vi "Error Handler.vi"(8 "Error code":T1=enum."5005: Path Type Not Supported") -> (0 "error out":errorcluster)   [LabVIEW 2016, in "LV-Data.PGSQL.lvclass"]
uses:
  LV-Data.PGSQL.lvclass
  Typedefs/Errors--enum.ctl
  <vilib>/Utility/error.llb/Error Cluster From Error Code.vi
  <vilib>/ErrorRing/Error Ring.xnode
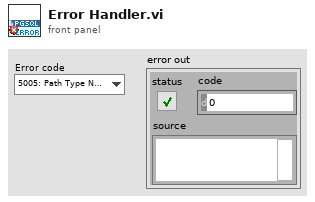
[diagram p1: front panel]
types:
  T1 = typedef "LV-Data.PGSQL.lvclass/Errors--enum.ctl" = enum16{"0: None", "5005: Path Type Not Supported", "5006: Number of Variables", "5008: Cannot write two data points", "5030: Start and End Times Identical", "5031: Input is not wholly", "5033: Bad path or paths", "5040: Invalid Instrument Name", "5050: Column can only hold string", "5051: Column can only hold bool", "5052: Column can only hold double", "5053: Column can only hold int"}
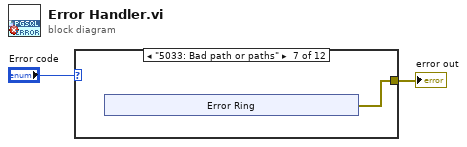
[diagram p0: block diagram]
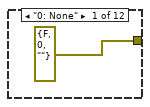
[diagram p2: hidden frame]
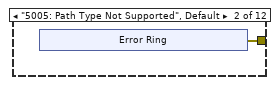
[diagram p3: hidden frame]
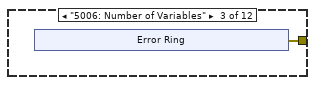
[diagram p4: hidden frame]
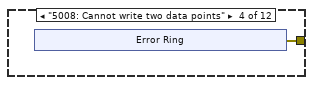
[diagram p5: hidden frame]
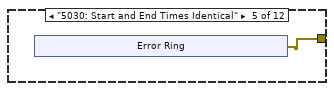
[diagram p6: hidden frame]
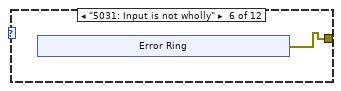
[diagram p7: hidden frame]
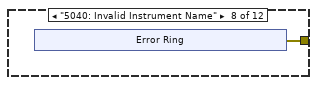
[diagram p8: hidden frame]
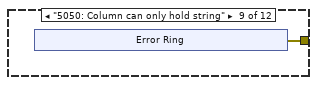
[diagram p9: hidden frame]
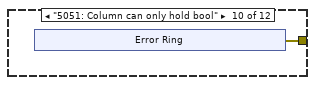
[diagram p10: hidden frame]
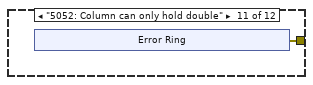
[diagram p11: hidden frame]
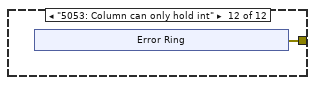
[diagram p12: hidden frame]
diagram:
  n1 = case shown="\"5033: Bad path or paths\"" "Error code" {
    tunnel: [errorcluster {"status"=FALSE, "code"=0, "source"=""} ("error out") w4 w10 w16 w22 w28 w34 w40 w46 w52 w58 w64] -> w1
    frame "0: None" {
    }
    frame "5005: Path Type Not Supported", Default {
      n2 = xnode "Error Ring"() -> ("error out"=w4:errorcluster)
    }
    frame "5006: Number of Variables" {
      n3 = xnode "Error Ring"() -> ("error out"=w10:errorcluster)
    }
    frame "5008: Cannot write two data points" {
      n4 = xnode "Error Ring"() -> ("error out"=w16:errorcluster)
    }
    frame "5030: Start and End Times Identical" {
      n5 = xnode "Error Ring"() -> ("error out"=w22:errorcluster)
    }
    frame "5031: Input is not wholly" {
      n6 = xnode "Error Ring"() -> ("error out"=w28:errorcluster)
    }
    frame "5033: Bad path or paths" {
      n7 = xnode "Error Ring"() -> ("error out"=w34:errorcluster)
    }
    frame "5040: Invalid Instrument Name" {
      n8 = xnode "Error Ring"() -> ("error out"=w40:errorcluster)
    }
    frame "5050: Column can only hold string" {
      n9 = xnode "Error Ring"() -> ("error out"=w46:errorcluster)
    }
    frame "5051: Column can only hold bool" {
      n10 = xnode "Error Ring"() -> ("error out"=w52:errorcluster)
    }
    frame "5052: Column can only hold double" {
      n11 = xnode "Error Ring"() -> ("error out"=w58:errorcluster)
    }
    frame "5053: Column can only hold int" {
      n12 = xnode "Error Ring"() -> ("error out"=w64:errorcluster)
    }
  }
  "error out" <- w1
